vi "Set Line Frequency.vi"(0 "VISA resource name":refnum<visa-resource-name>, 1 "Auto Frequency Detection (T: Enable)":bool=TRUE, 5 "Line Frequency (0: 60 Hz)":u16(ring) items=["60 Hz", "50 Hz"], 11 "error in (no error)":errorcluster) -> (4 "VISA resource name out":refnum<visa-resource-name>, 15 "error out":errorcluster)   [LabVIEW 2024, in "Keithley 648X Series.lvlib"]
doc: "Sets the operating power line frequency of the instrument."
uses:
  <instrlib>/Keithley 648X Series/Keithley 648X Series.lvlib
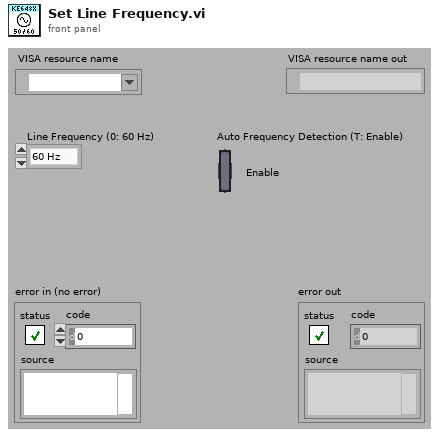
[diagram p1: front panel]
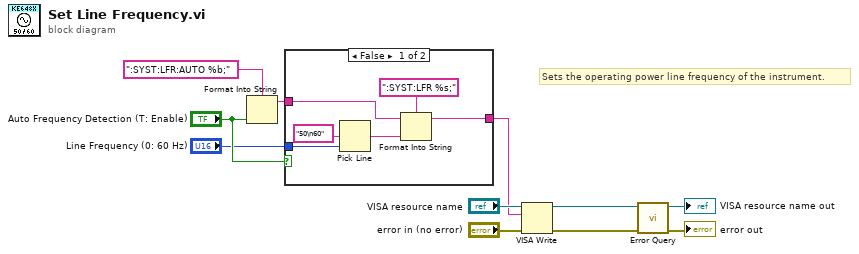
[diagram p0: block diagram]
diagram:
  # "Sets the operating power line frequency of the instrument."
  n1 = Format Into String(format string=":SYST:LFR:AUTO %b;", "Auto Frequency Detection (T: Enable)") -> (resulting string=w3:string)  [unwired: 2 in, 1 out]
  n2 = case shown="False" "Auto Frequency Detection (T: Enable)" {
    tunnel: w3 -> [w13 w18]
    tunnel: [w12 w18] -> w2
    tunnel: "Line Frequency (0: 60 Hz)" -> [w17 _]
    frame False {
      n3 = Pick Line(multi-line string="50\n60", line index=w17) -> (output string=w15:string)  [unwired: 1 in]
      n4 = Format Into String(format string=":SYST:LFR %s;", initial string=w13, w15) -> (resulting string=w12:string)  [unwired: 1 in, 1 out]
    }
    frame True {
    }
  }
  n5 = VISA Write(VISA resource name="VISA resource name", write buffer=w2, error in (no error)="error in (no error)") -> (VISA resource name out=w8:refnum<visa-resource-name>, error out=w9:errorcluster)  [unwired: 1 out]
  n6 = call <instrlib>:"Error Query.vi"("error in (no error)"=w9, "VISA resource name"=w8) -> ("error out"=→"error out":errorcluster, "VISA resource name out"=→"VISA resource name out":refnum<visa-resource-name>)  [unwired: 6 in, 2 out]
